vi "niDTS BT EDR Tx Test Configure.vi"(0 "Dummy Test Handle In":T10, 7 "EDR Tx Input Parameters":T1={"Channel"=3, "Dut Tx Power  (dBm)"=0.0, "Auto Level"=FALSE, "External Attenuation (dB)"=0.0, "EDR Packet type"=enum."DH1", "Data Rate"=2, "Payload Data"=enum."PN9", "Burst Sync"=enum."PREamble", "Packet Length, bytes"=-1, "BD ADDRESS"="", "Trace Enable"=FALSE, "EDR ModAcc Measurement"={"DEVM Enable"=FALSE, "Averages"=1, "Averaging Mode"=enum."RMS", "Measurement Duration (bytes)"=-1, "Measurement Offset (bytes)"=0}, "TXP Measurement"={"TXP Power Enable"=FALSE, "TXP Averages"=1, "Averaging Type"=enum."RMS"}, "IBE  Measurement"={"IBE Enable"=FALSE, "IBE Averages"=1, "Averaging Type"=enum."RMS", "Numbe of Channels"=11, "Channel Mode"=enum."Centered", "Measurement Interval Mode"=enum."AUTO", "Measurement Interval Length (sec)"=0.005}, "Trigger"={"MinQuietTimeDuration (sec)"=0.0001, "TriggerDelay (sec)"=0.0, "TriggerEdge"=enum."RISing", "TriggerSource"=enum."RF0", "TriggerThreshold (dB)"=20.0, "TriggerTimeout (sec)"=10.0}} {"Trigger"."MinQuietTimeDuration (sec)" format="%#_6p"; "Data Rate" min=2 max=3 step=1}, 9 "ResultsIndex":u8=1, 11 "error in (no error)":errorcluster) -> (4 "Dummy Test Handle Out":T10, 15 "error out":errorcluster)   [LabVIEW 2014, in "niDTS BT.lvlib"]
uses:
  niDTS BT.lvlib
  Tx Test/Includes/niDTS BT Tx Test INC Handle.ctl
  Tx Test/Objects/BASE_class/niDTS BT Tx Test.lvclass
  Includes/niDTS BT EDR Tx Test INC Parameters.ctl
  Includes/niDTS BT INC EDR Packet Type.ctl
  Includes/niDTS BT INC EDR Data Rate.ctl
  Tx Test/Includes/niDTS BT Tx Test INC BD Payload Data.ctl
  Includes/niDTS BT INC EDR Burst Sync.ctl
  Includes/niDTS BT INC EDR ModAcc Measurement Parameters.ctl
  Includes/niDTS BT INC TXP Measurement Parameters.ctl
  Includes/niDTS BT INC EDR IBE Measurement Parameters.ctl
  Includes/niDTS BT DUT INC Trigger.ctl
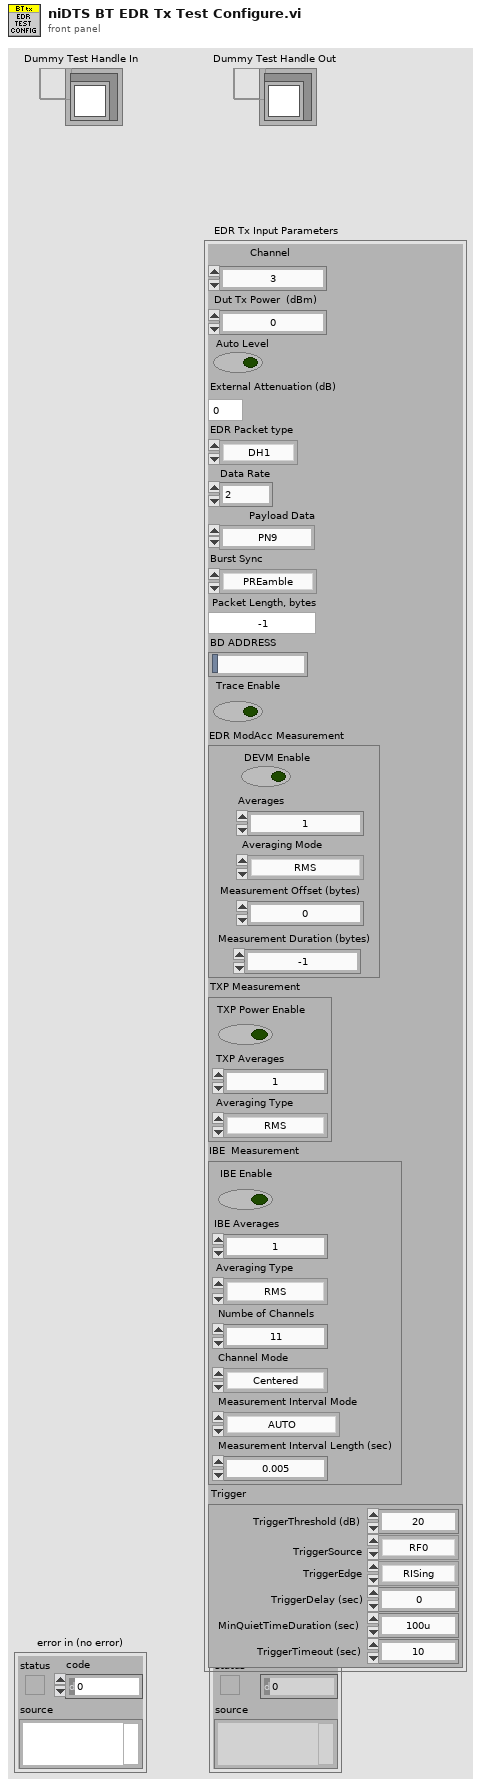
[diagram p1: front panel]
types:
  T1 = typedef "niDTS BT.lvlib/niDTS BT EDR Tx Test INC Parameters.ctl" = cluster{"Channel":i32, "Dut Tx Power  (dBm)":dbl, "Auto Level":bool, "External Attenuation (dB)":dbl, "EDR Packet type":T2, "Data Rate":T3, "Payload Data":T4, "Burst Sync":T5, "Packet Length, bytes":i32, "BD ADDRESS":string, "Trace Enable":bool, "EDR ModAcc Measurement":T6, "TXP Measurement":T7, "IBE  Measurement":T8, "Trigger":T9}
  T2 = typedef "niDTS BT.lvlib/niDTS BT INC EDR Packet Type.ctl" = enum16{"NULL", "POLL", "FHS", "DM1", "DH1", "HV1", "HV2", "HV3", "EV3", "DV", "AUX1", "DM3", "DH3", "EV4", "EV5", "DM5", "DH5"}
  T3 = typedef "niDTS BT.lvlib/niDTS BT INC EDR Data Rate.ctl" = i32
  T4 = typedef "niDTS BT.lvlib/niDTS BT Tx Test INC BD Payload Data.ctl" = enum16{"0", "1", "01", "00001111", "PN9", "AUTO"}
  T5 = typedef "niDTS BT.lvlib/niDTS BT INC EDR Burst Sync.ctl" = enum16{"NONE", "PREamble"}
  T6 = typedef "niDTS BT.lvlib/niDTS BT INC EDR ModAcc Measurement Parameters.ctl" = cluster{"DEVM Enable":bool, "Averages":i32, "Averaging Mode":enum16{"RMS", "LOG", "SCALAR", "MAX", "MIN", "VECTOR"}, "Measurement Duration (bytes)":i32, "Measurement Offset (bytes)":i32}
  T7 = typedef "niDTS BT.lvlib/niDTS BT INC TXP Measurement Parameters.ctl" = cluster{"TXP Power Enable":bool, "TXP Averages":i32, "Averaging Type":enum16{"RMS", "LOG", "SCALAR", "MAX", "MIN"}}
  T8 = typedef "niDTS BT.lvlib/niDTS BT INC EDR IBE Measurement Parameters.ctl" = cluster{"IBE Enable":bool, "IBE Averages":i32, "Averaging Type":enum16{"RMS", "LOG", "SCALAR", "MAX", "MIN", "VECTOR"}, "Numbe of Channels":i32, "Channel Mode":enum16{"InBand", "Centered"}, "Measurement Interval Mode":enum16{"AUTO", "MANUAL"}, "Measurement Interval Length (sec)":dbl}
  T9 = typedef "niDTS BT.lvlib/niDTS BT DUT INC Trigger.ctl" = cluster{"MinQuietTimeDuration (sec)":dbl, "TriggerDelay (sec)":dbl, "TriggerEdge":enum16{"RISing", "FALLing"}, "TriggerSource":enum16{"IMMediate", "RF0", "PFI0", "PFI1", "RTS0", "RTS1", "RTS2", "RTS3", "RTS4", "RTS5", "RTS6", "RTS7", "PXIStar", "SOFT"}, "TriggerThreshold (dB)":dbl, "TriggerTimeout (sec)":dbl}
  T10 = typedef "niDTS BT.lvlib/niDTS BT Tx Test INC Handle.ctl" = refnum<data-value>
  T11 = typedef "niDTS BT.lvlib/niDTS BT Tx Test INC Parameters.ctl" = cluster{"Channel":i32, "Data Rate ":i32, "Dut Tx Power":dbl, "External Attenuation (dB)":dbl[], "Auto Level":bool, "Packet type":T12, "Payload Pattern":T4, "Burst Sync":enum16{"NONE", "PREamble"}, "BD ADDRESS":u32, "Packet Length, bytes":i32, "ModAcc Measurement Paramaters":cluster{"ModAcc Enable":bool, "CFO Enable":bool, "Character Select":T13, "Averages":i32, "Averaging Mode":enum16{"RMS", "LOG", "SCALAR", "MAX", "MIN", "VECTOR"}, "Measurement Length":i32, "Measurement Offset":i32}, "OBW Measurement Parameters":T14, "TXP Measurement Parameters":T7, "IBE  Measurement Parameters":T8, "Trace Enable":bool, "Trigger":T9}
  T12 = typedef "niDTS BT.lvlib/niDTS BT INC Packet Type.ctl" = enum16{"NULL", "POLL", "FHS", "DM1", "DH1", "HV1", "HV2", "HV3", "EV3", "DV", "AUX1", "DM3", "DH3", "EV4", "EV5", "DM5", "DH5", "LE-TP"}
  T13 = typedef "niDTS BT.lvlib/niDTS BT Tx Test INC Modulation Characteristics.ctl" = enum16{"DF1", "DF2", "BOTH"}
  T14 = typedef "niDTS BT.lvlib/niDTS BT INC OBW Measurement Parameters.ctl" = cluster{"OBW Enable":bool, "OBW Averages":i32, "Averaging Type":enum16{"RMS", "LOG", "SCALAR", "MAX", "MIN", "VECTOR"}, "Measurement Interval Mode":enum16{"AUTO", "MANUAL"}, "Measurement Interval Length (sec)":dbl}
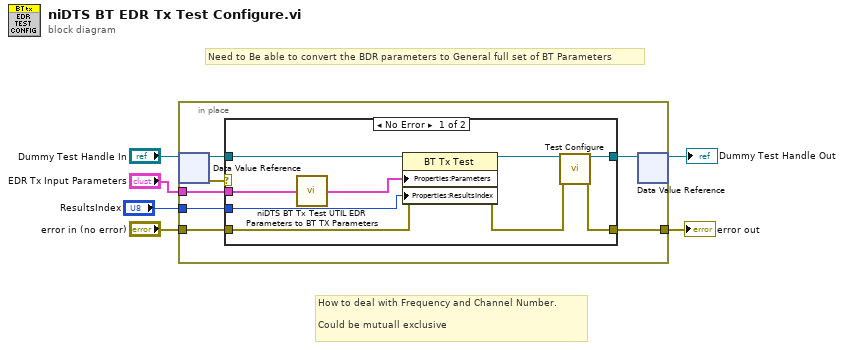
[diagram p0: block diagram]
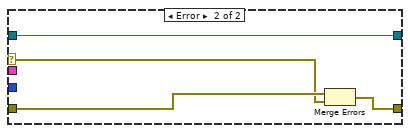
[diagram p2: hidden frame]
diagram:
  # "Need to Be able to convert the BDR parameters to General full set of BT Parameters"
  # "How to deal with Frequency and Channel Number.\n\nCould be mutuall exclusive"
  n1 = in-place {
    in-place-border: "error in (no error)" -> [w10]
    in-place-border: [w9] -> w5
    in-place-border: "EDR Tx Input Parameters" -> [w8]
    in-place-border: "ResultsIndex" -> [w7]
    n2 = in-place-dvr #1("Dummy Test Handle In") -> (w12:refnum<class "niDTS BT Tx Test.lvclass">, w13:errorcluster)
    n3 = case shown="No Error" w13 {
      selector: w13 -> [_ w24]
      tunnel: w12 -> [w22 w26]
      tunnel: [w18 w26] -> w11
      tunnel: w10 -> [w21 w25]
      tunnel: [w19 w23] -> w9
      tunnel: w8 -> [w14 _]
      tunnel: w7 -> [w16 _]
      frame No Error {
        n4 = call "niDTS BT Tx Test UTIL EDR Parameters to BT TX Parameters.vi"("EDR Tx Input Parameters"=w14) -> ("BT Tx Input Parameters"=w15:T11)  [unwired: 14 in]
        n5 = property class="BT Tx Test"(reference=w22, error in=w21, "Properties:Parameters"=w15, "Properties:ResultsIndex"=w16) -> (reference out=w17:refnum<class "niDTS BT Tx Test.lvclass">, error out=w20:errorcluster)
        n6 = call-dynamic "Test Configure.vi"("Template Tx Test in"=w17, "error in (no error)"=w20) -> ("Template Tx Test out"=w18:refnum<class "niDTS BT Tx Test.lvclass">, "error out"=w19:errorcluster)  [unwired: 12 in]
      }
      frame Error {
        n7 = Merge Errors(w25, w24) -> (w23:errorcluster)
      }
    }
    n8 = in-place-dvr #1(w11) -> (→"Dummy Test Handle Out":T10)  [unwired: 1 out]
  }
  "error out" <- w5
